vi "ZDataVIS_SimpleSliceDataToIntensity.vi"(4 "Y AXIS":i32(listbox), 5 "Z":T4(ring), 6 "X AXIS":i32(listbox), 7 "X":T4(ring), 8 "error in (no error)":errorcluster, 10 "Outer Indices":T1, 11 "Big Ol Array IN":T3(array[cluster])) -> (0 "error out":errorcluster, 2 "Intensity Graph":dbl[][](graph), 3 "Intensity Info OUT":cluster{dbl[], dbl[]}[](array[cluster]))   [LabVIEW 2016]
panel:
  out "x+y":i32
  in  "Slide":dbl(slide) scale=0.0..250.0
  in  "Inner Indices":dbl[](array[numeric])
  in  "Cursor Z index":i32
  in  "Cursor Y index":i32
  in  "Cursor X index":i32
  in  "Cursor Graph Z Variable":T2(ring)=enum."Vslowestest"
  in  "Cursor Graph Y Variable":T2(ring)=enum."Vslowestest"
  in  "Cursor Graph X Variable":T2(ring)=enum."Vslowestest"
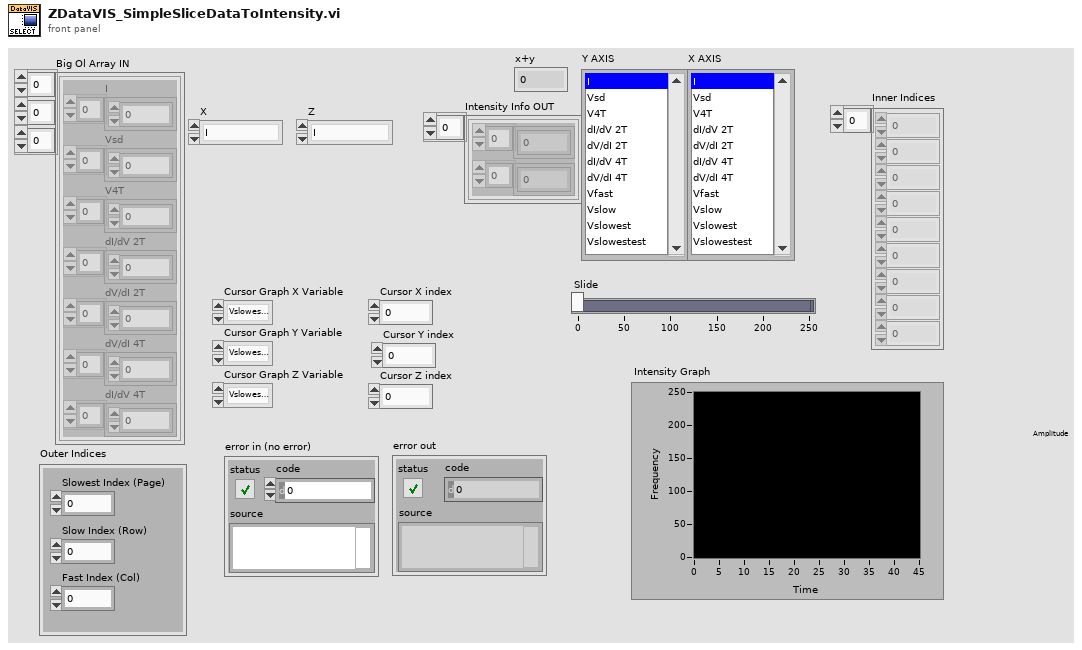
[diagram p1: front panel]
types:
  T1 = cluster{"Slow Index (Row)":dbl, "Slowest Index (Page)":i32, "Fast Index (Col)":i32}
  T2 = enum16{"Vfast", "Vslow", "Vslowest", "Vslowestest"}
  T3 = cluster{"I":dbl[], "Vsd":dbl[], "V4T":dbl[], "dI/dV 2T":dbl[], "dV/dI 2T":dbl[], "dV/dI 4T":dbl[], "dI/dV 4T":dbl[]}[][][]
  T4 = enum16{"I", "Vsd", "V4T", "dI/dV 2T", "dV/dI 2T", "dV/dI 4T", "dI/dV 4T"}
  T5 = cluster{"I":dbl[], "Vsd":dbl[], "V4T":dbl[], "dI/dV 2T":dbl[], "dV/dI 2T":dbl[], "dV/dI 4T":dbl[], "dI/dV 4T":dbl[]}[][]
  T6 = cluster{"I":dbl[], "Vsd":dbl[], "V4T":dbl[], "dI/dV 2T":dbl[], "dV/dI 2T":dbl[], "dV/dI 4T":dbl[], "dI/dV 4T":dbl[]}[]
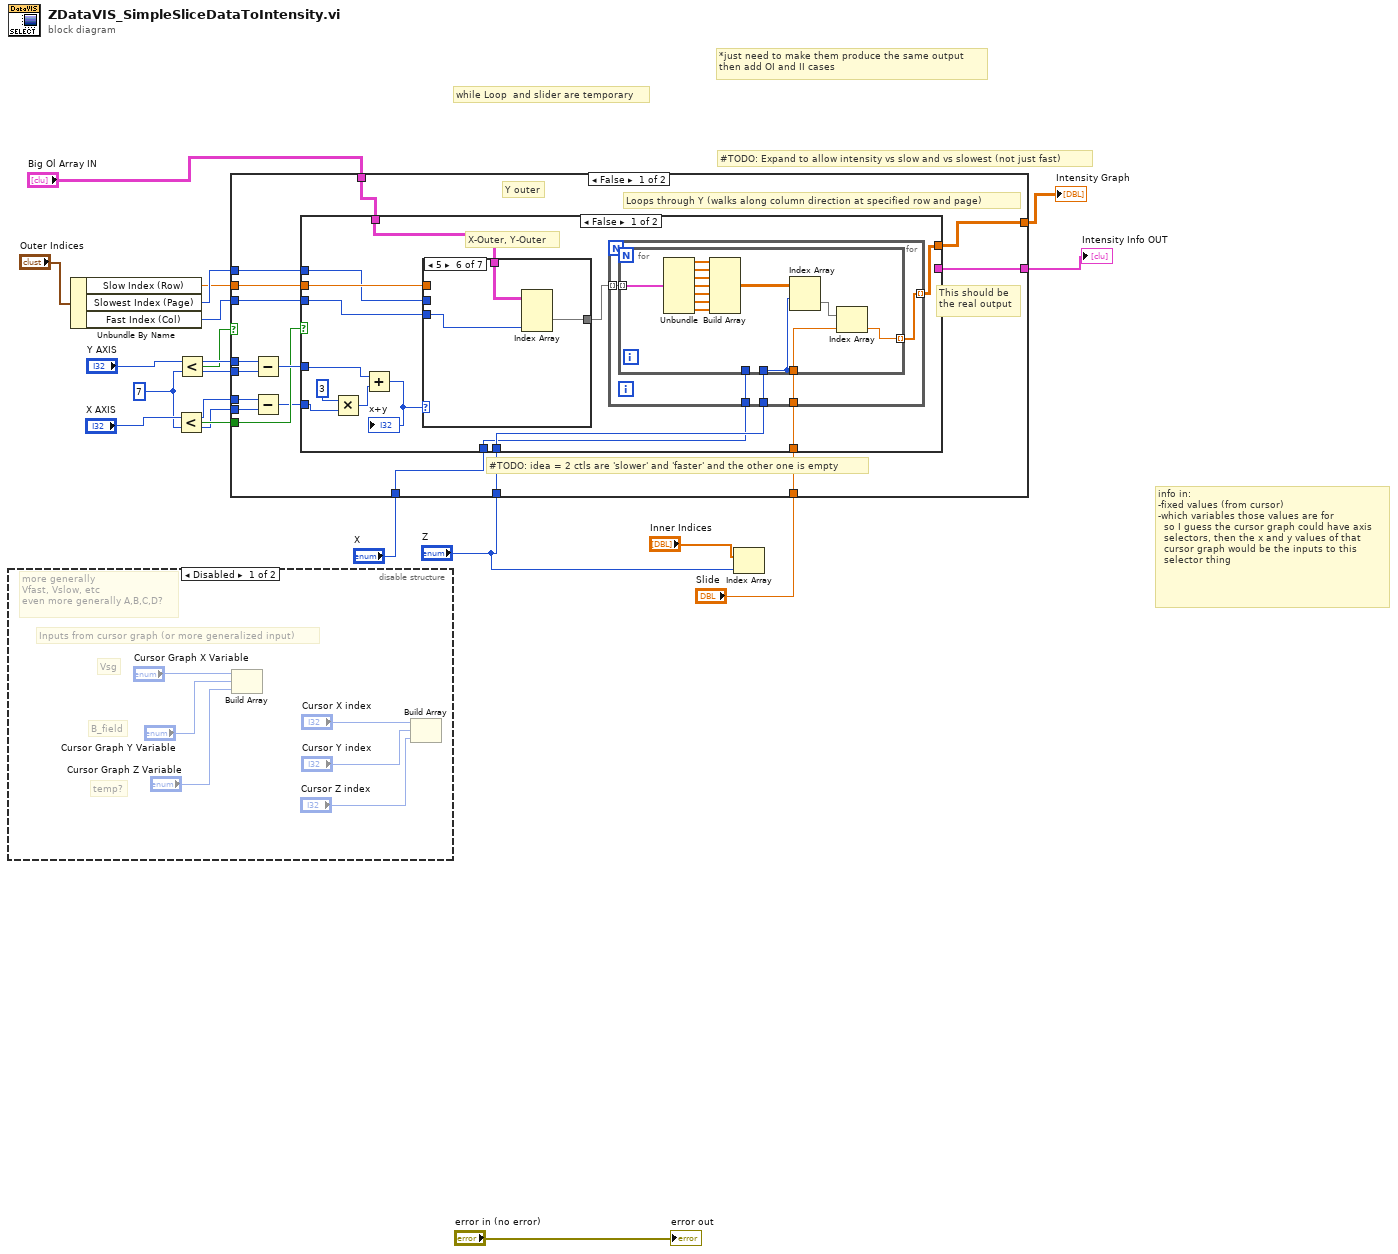
[diagram p0: block diagram]
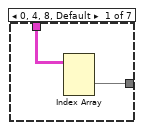
[diagram p2: hidden frame]
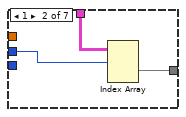
[diagram p3: hidden frame]
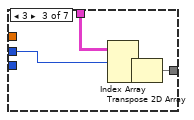
[diagram p4: hidden frame]
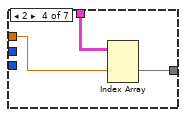
[diagram p5: hidden frame]
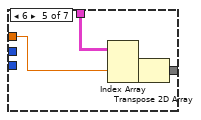
[diagram p6: hidden frame]
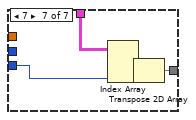
[diagram p7: hidden frame]
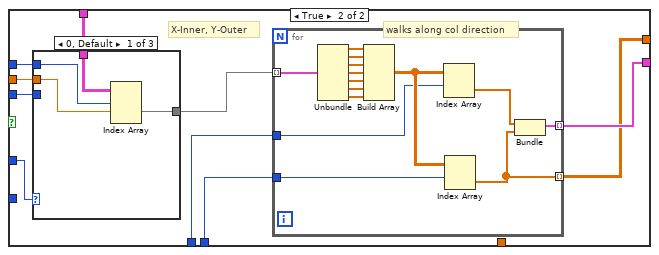
[diagram p8: hidden frame]
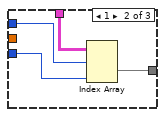
[diagram p9: hidden frame]
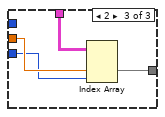
[diagram p10: hidden frame]
diagram:
  w8 = 7 ("y")
  # "info in:\n-fixed values (from cursor)\n-which variables those values are for\n  so I guess the cursor graph could have axis\n  selectors, then the x and y values of that \n  cursor graph would be the inputs to this\n  selector thing"
  # "#TODO: Expand to allow intensity vs slow and vs slowest (not just fast)"
  # "*just need to make them produce the same output\nthen add OI and II cases"
  # "while Loop  and slider are temporary"
  n1 = disable-structure shown="Disabled" {
    frame Disabled {
      # "more generally\nVfast, Vslow, etc\neven more generally A,B,C,D?"
      # "temp?"
      # "B_field"
      # "Vsg"
      # "Inputs from cursor graph (or more generalized input)"
      n2 = Build Array("Cursor Graph X Variable", "Cursor Graph Y Variable", "Cursor Graph Z Variable") -> ()  [unwired: 1 out]
      n3 = Build Array("Cursor X index", "Cursor Y index", "Cursor Z index") -> ()  [unwired: 1 out]
    }
    frame Enabled {
    }
  }
  n4 = Unbundle By Name("Outer Indices") -> ("Slow Index (Row)"=w14:dbl, "Slowest Index (Page)"=w15:i32, "Fast Index (Col)"=w13:i32)
  n5 = Less?(x="X AXIS", y=w8) -> (x < y?=w10:bool)
  n6 = Less?(x="Y AXIS", y=w8) -> (x < y?=w11:bool)
  n7 = case shown="False" w11 {
    tunnel: [w28 _] -> w6
    tunnel: "Big Ol Array IN" -> [w39 _]
    tunnel: w15 -> [w38 _]
    tunnel: w14 -> [w37 _]
    tunnel: w13 -> [w36 _]
    tunnel: "Y AXIS" -> [w34 _]
    tunnel: w8 -> [w35 _]
    tunnel: w10 -> [w32 _]
    tunnel: "X AXIS" -> [w31 _]
    tunnel: w8 -> [w30 _]
    tunnel: "X" -> [w27 _]
    tunnel: "Z" -> [w26 _]
    tunnel: [w24 _] -> w2
    tunnel: "Slide" -> [w25 _]
    frame False {
      # "This should be \nthe real output"
      # "Y outer"
      # "Loops through Y (walks along column direction at specified row and page)"
      # "#TODO: idea = 2 ctls are 'slower' and 'faster' and the other one is empty"
      n8 = Subtract(x=w34, y=w35) -> (x-y=w33:i32)
      n9 = Subtract(x=w31, y=w30) -> (x-y=w29:i32)
      n10 = case shown="False" w32 {
        tunnel: [w44 w95] -> w28
        tunnel: w39 -> [w53 w103]
        tunnel: w38 -> [w47 w102]
        tunnel: w37 -> [w48 w101]
        tunnel: w36 -> [w46 w100]
        tunnel: w33 -> [w49 w99]
        tunnel: w29 -> [w52 _]
        tunnel: w27 -> [w40 w98]
        tunnel: w26 -> [w43 w97]
        tunnel: [_ w96] -> w24
        tunnel: w25 -> [w41 _]
        frame False {
          # "X-Outer, Y-Outer"
          n11 = Multiply(x=3, y=w52) -> (x*y=w50:i32)
          n12 = Add(x=w49, y=w50) -> (x+y=w42:i32)
          "x+y" <- w42
          n13 = case shown="5" w42 {
            tunnel: [w72 w74 w77 w82 w84 w89 w91] -> w45
            tunnel: w53 -> [w73 w76 w79 w83 w87 w90 w94]
            tunnel: w47 -> [_ w75 w78 _ _ _ _]
            tunnel: w48 -> [_ _ _ w81 w85 _ _]
            tunnel: w46 -> [_ _ _ _ _ w88 w92]
            frame 0, 4, 8, Default {
              n14 = Index Array(array=w73) -> (element=w72:T5)  [unwired: 3 in]
            }
            frame 1 {
              n15 = Index Array(array=w76, index (dim 0)=w75) -> (element=w74:T5)  [unwired: 2 in]
            }
            frame 3 {
              n16 = Index Array(array=w79, index (dim 0)=w78) -> (element=w80:T5)  [unwired: 2 in]
              n17 = Transpose 2D Array(2D array=w80) -> (transposed array=w77:T5)
            }
            frame 2 {
              n18 = Index Array(array=w83, index (dim 1)=w81) -> (element=w82:T5)  [unwired: 2 in]
            }
            frame 6 {
              n19 = Index Array(array=w87, index (dim 1)=w85) -> (element=w86:T5)  [unwired: 2 in]
              n20 = Transpose 2D Array(2D array=w86) -> (transposed array=w84:T5)
            }
            frame 5 {
              n21 = Index Array(array=w90, index (dim 2)=w88) -> (element=w89:T5)  [unwired: 2 in]
            }
            frame 7 {
              n22 = Index Array(array=w94, index (dim 2)=w92) -> (element=w93:T5)  [unwired: 2 in]
              n23 = Transpose 2D Array(2D array=w93) -> (transposed array=w91:T5)
            }
          }
          n24 = for {
            tunnel: w45 -> [w58] mode=indexing
            tunnel: [w57] -> w44 mode=indexing
            tunnel: w43 -> [w56]
            tunnel: w41 -> [w55]
            tunnel: w40 -> [w54]
            n25 = for {
              tunnel: w58 -> [w64] mode=indexing
              tunnel: [w60] -> w57 mode=indexing
              tunnel: [w62] -> _ mode=indexing
              tunnel: w56 -> [w62]
              tunnel: w55 -> [w59]
              tunnel: w54 -> [_]
              n26 = Unbundle(w64) -> ("I"=w71:dbl[], "Vsd"=w70:dbl[], "V4T"=w69:dbl[], "dI/dV 2T"=w68:dbl[], "dV/dI 2T"=w67:dbl[], "dV/dI 4T"=w66:dbl[], "dI/dV 4T"=w65:dbl[])
              n27 = Build Array(w71, w70, w69, w68, w67, w66, w65) -> (w63:dbl[][])
              n28 = Index Array(array=w63, index (row)=w62) -> (element=w61:dbl[])  [unwired: 1 in]
              n29 = Index Array(array=w61, index=w59) -> (element=w60:dbl)
            }
          }
        }
        frame True {
          # "walks along col direction"
          # "X-Inner, Y-Outer"
          n30 = case shown="0, Default" w99 {
            tunnel: w102 -> [w106 w112 _]
            tunnel: [w107 w111 w113] -> w104
            tunnel: w101 -> [w105 _ w115]
            tunnel: w103 -> [w108 w110 w116]
            tunnel: w100 -> [_ w109 w114]
            frame 0, Default {
              n31 = Index Array(array=w108, index (dim 0)=w106, index (dim 1)=w105) -> (element=w107:T6)  [unwired: 1 in]
            }
            frame 1 {
              n32 = Index Array(array=w110, index (dim 0)=w112, index (dim 2)=w109) -> (element=w111:T6)  [unwired: 1 in]
            }
            frame 2 {
              n33 = Index Array(array=w116, index (dim 1)=w115, index (dim 2)=w114) -> (element=w113:T6)  [unwired: 1 in]
            }
          }
          n34 = for {
            tunnel: w104 -> [w123] mode=indexing
            tunnel: [w120] -> w96 mode=indexing
            tunnel: w98 -> [w119]
            tunnel: w97 -> [w118]
            tunnel: [w117] -> w95 mode=indexing
            n35 = Unbundle(w123) -> ("I"=w130:dbl[], "Vsd"=w129:dbl[], "V4T"=w128:dbl[], "dI/dV 2T"=w127:dbl[], "dV/dI 2T"=w126:dbl[], "dV/dI 4T"=w125:dbl[], "dI/dV 4T"=w124:dbl[])
            n36 = Build Array(w130, w129, w128, w127, w126, w125, w124) -> (w122:dbl[][])
            n37 = Index Array(array=w122, index (row)=w119) -> (element=w121:dbl[])  [unwired: 1 in]
            n38 = Index Array(array=w122, index (row)=w118) -> (element=w117:dbl[])  [unwired: 1 in]
            n39 = Bundle(w121, w117) -> (w120:cluster{dbl[], dbl[]})  [unwired: 1 in]
          }
        }
      }
    }
    frame True {
      # "Y inner"
    }
  }
  "Intensity Graph" <- w6
  "Intensity Info OUT" <- w2
  n40 = Index Array(array="Inner Indices", index="Z") -> ()  [unwired: 1 out]
  "error out" <- "error in (no error)"
